vi "tip_light_error.vi"() -> (0 "Residues":dbl[][][](array[numeric]) format="%#.0f", 3 "RMS error":dbl[](array[numeric]) format="%#.0f")   [LabVIEW 2014]
uses:
  initialization/micron_globals.vi
  <vilib>/Analysis/Matrix/Numeric/Conversions/Array To Matrix - RA2.vi
  <vilib>/Analysis/Matrix/NI_Matrix.lvlib
panel:
  # "Find the error of pose estimation according to the mismatch between the measured light positions + pose and the calibrated positions."
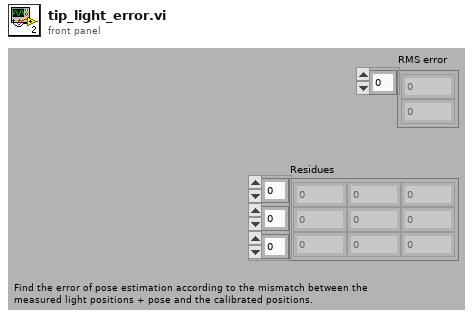
[diagram p1: front panel]
types:
  T1 = typedef "Micron params.ctl" = cluster{"Stimulus":T2, "Goal Filter A":T4, "Mode controls":T5, "Manipulator type":enum16{"Current piezo", "Voltage piezo"}, "Manipulator calibration":T6, "Network":T8, "Goal Filter B":T4, "Cancellation":T9, "Transition time":sgl, "Estimation":T11}
  T2 = typedef "stimulus.ctl" = cluster{"Type":enum16{"Off", "Step", "Sine", "Triangle", "Arbitrary"}, "Phase":dbl, "Amplitude":sgl[], "Injection point":T3, "Closed loop":bool, "Offset":sgl[], "Tip -> world":bool, "Frequency":dbl, "Length":dbl}
  T3 = typedef "injection_point.ctl" = enum16{"Total pose", "V limiter", "Goal ", "Link position", "KF link position", "Inverse kin", "Link goal", "Link error", "Controller", "Output", "Drive", "Light"}
  T4 = typedef "goal_loop_parms.ctl" = cluster{"Speedup max":sgl, "Speedup thresh":sgl, "Speedup nonlin":sgl, "Filters":cluster{"Lower Fc":sgl, "Lower Q":sgl, "Scale factor":sgl, "Upper Fc":sgl, "Upper Q":sgl, "V limit":sgl, "V limit range":sgl}[]}
  T5 = typedef "mode_conrols.ctl" = cluster{"Hold":bool, "Cancellation":bool, "Goal filter":bool, "Trigger":bool}
  T6 = typedef "manipulator_cal.ctl" = cluster{"Tool offsets":sgl[][], "Handle light calibration":T7, "Base pivots":sgl[][], "Output pivots":sgl[][], "Length center":sgl, "Workspace height":sgl[], "Workspace diameter":sgl[], "Stack travel":sgl, "Saturation pos":sgl, "Inverse filters":cluster{"filter structure":enum32{"IIR 2nd Order", "IIR 4th Order"}, "Reverse Coefficients":dbl[], "Forward Coefficients":dbl[]}[], "Strut length":sgl, "Tip light calibration":T7}
  T7 = typedef "probe_calibration.ctl" = sgl[][]
  T8 = typedef "network_params.ctl" = cluster{"Remote Host":string, "Send Status":bool, "Send Port":u16, "Recv Commands":bool, "Recv Port":u16}
  T9 = typedef "sq_control_params.ctl" = cluster{"KP":T10, "KI":sgl, "KD":T10, "Max vel":sgl, "Max acc":sgl, "Int error limit":sgl, "RCM gain":sgl, "Bypass":bool, "Degraded gain":sgl}
  T10 = typedef "decoupled_gain.ctl" = cluster{"XY":sgl, "Rxy":sgl, "Z":sgl, "Rz":sgl}
  T11 = typedef "estimation_controls.ctl" = cluster{"Link":cluster{"Measure noise":dbl[], "Process noise":dbl[], "Alt process noise":dbl[], "Alt turnoff cycles":i32, "Innovation limit":dbl[], "Residue threshold":dbl, "Enable":bool}, "Handle":cluster{"Measure noise":dbl[], "Process noise":dbl[], "State limits":dbl[], "Innovation limit":dbl[], "Prediction Lookahead":sgl, "Enable":bool}}
  T12 = typedef "NI_Matrix.lvlib/RealMatrix.ctl" = dbl[][]
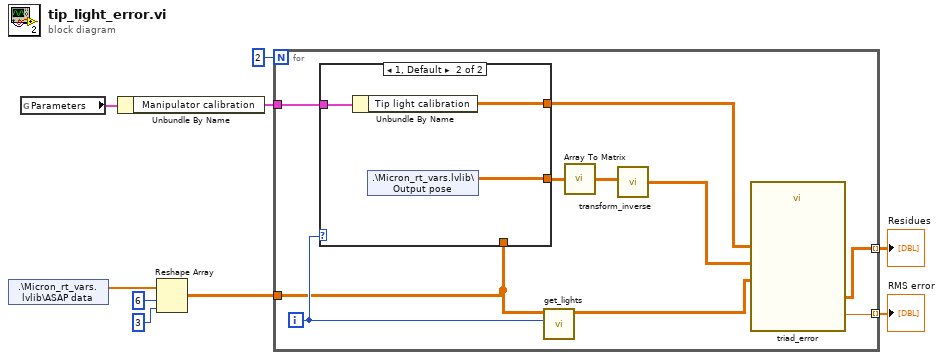
[diagram p0: block diagram]
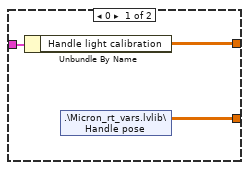
[diagram p2: hidden frame]
diagram:
  n1 = shared-variable ".\\Micron_rt_vars.lvlib\\ASAP data"() -> (w1:sgl[])  [unwired: 2 out]
  n2 = global read "micron_globals.vi" "Parameters"() -> (w8:T1)
  n3 = Unbundle By Name(w8) -> ("Manipulator calibration"=w9:T6)
  n4 = Reshape Array(w1, 6 ("dimension size"), 3 ("dimension size")) -> (w4:sgl[][])
  n5 = for {
    N: 2 -> [_]
    tunnel: w9 -> [w19]
    tunnel: [w15] -> w6 mode=indexing
    tunnel: [w13] -> w5 mode=indexing
    tunnel: w4 -> [w10]
    i -> [w16]
    n6 = case shown="1, Default" w16 {
      tunnel: w19 -> [w22 w25]
      tunnel: [w21 w23] -> w18
      tunnel: [w20 w24] -> w17
      tunnel: w10 -> [_ _]
      frame 0 {
        n7 = Unbundle By Name(w22) -> ("Handle light calibration"=w21:T7)
        n8 = shared-variable ".\\Micron_rt_vars.lvlib\\Handle pose"() -> (w20:sgl[][])  [unwired: 2 out]
      }
      frame 1, Default {
        n9 = Unbundle By Name(w25) -> ("Tip light calibration"=w23:T7)
        n10 = shared-variable ".\\Micron_rt_vars.lvlib\\Output pose"() -> (w24:sgl[][])  [unwired: 2 out]
      }
    }
    n11 = call "get_lights.vi"("Selector"=w16, "ASAP data"=w10) -> ("Light positions"=w14:T7)  [unwired: 9 in]
    n12 = call-poly <vilib>:"Array To Matrix.vi"("Real 2D Array"=w17) -> ("Real Matrix"=w12:T12)
    n13 = call "transform_inverse.vi"("Transform"=w12) -> ("Inverse transform"=w11:T12)
    n14 = call "triad_error.vi"("Measured positions"=w14, "Measure transform"=w11, "Calibrated positions"=w18) -> ("Residues"=w15:T7, "RMS error"=w13:dbl)  [unwired: 7 in]
  }
  "Residues" <- w6
  "RMS error" <- w5
